vi "PM100D_Write.vi"(2 "error in (no error)":errorcluster, 3 "Command":string, 4 "VISA in":refnum<visa-resource-name>="COM1") -> (0 "error out":errorcluster, 1 "VISA out":refnum<visa-resource-name>)   [LabVIEW 2016]
doc: "Writes a SCPI command to the connected instrument"
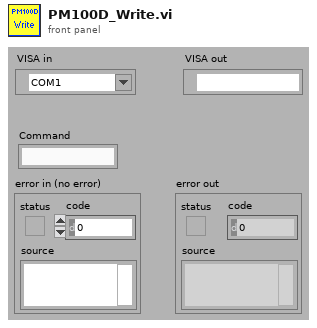
[diagram p1: front panel]
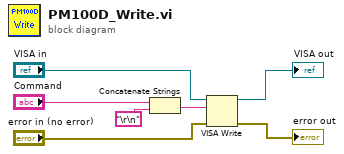
[diagram p0: block diagram]
diagram:
  n1 = Concatenate Strings("Command", "\r\n") -> (w7:string)
  n2 = VISA Write(VISA resource name="VISA in", write buffer=w7, error in (no error)="error in (no error)") -> (VISA resource name out=→"VISA out":refnum<visa-resource-name>, error out=→"error out":errorcluster)  [unwired: 1 out]
